vi "Cycle.vi"(8 "error in (no error)":errorcluster, 11 "WhiteNoiseOrientationDetection In":refnum<class "WhiteNoiseOrientationDetection.lvclass">) -> (0 "error out":errorcluster, 3 "WhiteNoiseOrientationDetection Out":refnum<class "WhiteNoiseOrientationDetection.lvclass">)   [LabVIEW 2014, in "WhiteNoiseOrientationDetection.lvclass"]
uses:
  WhiteNoiseOrientationDetection.lvclass
  WhiteNoiseOrientationDetection.lvclass/WhiteNoiseOrientationDetection.ctl
  Trial Based Experiment Statechart/MatlabExperiment/MatlabExperiment.lvclass
panel:
  in  "Override location":bool
  in  "location":dbl=1.0 max=10000.0
  in  "ExtraReward":dbl=0.8 min=0.0 step=0.1 format="%.1g"
  in  "Intertrial":dbl=1300.0
  in  "Override Coherence":bool
  in  "Override Signal":bool
  in  "Override Catch Trial":bool
  in  "coherence":dbl=35.0 max=10000.0
  in  "signal":dbl=135.0 max=10000.0
  in  "Override Timing":bool
  in  "PunishTime":dbl=2900.0
  out "InResponseWindow":bool
  in  "targetFixationRadius":dbl=75.0
  in  "nFramesCohTrain":dbl=50.0
  in  "nFramesPreMaxTrain":dbl=400.0
  in  "nFramesPreMeanTrain":dbl=150.0
  in  "nFramesPreMinTrain":dbl=100.0
  in  "responseIntervalTrain":dbl=50.0 max=10000.0
  in  "Eye Params":dbl[](array[numeric])
  out "XY Graph":cluster{dbl[], dbl[]}(graph)
  in  "MinReward":dbl=35.0
  in  "FixationRadius":dbl=50.0
  out "Timeouts":T1={"Intertrial"=1000.0, "AcquireFixation"=1000.0, "HoldFixation"=300.0, "DelayPeriod"=1000.0, "ResponsePeriod"=1000.0}
  out "ExperimentStats":T2
  out "Cycles":dbl
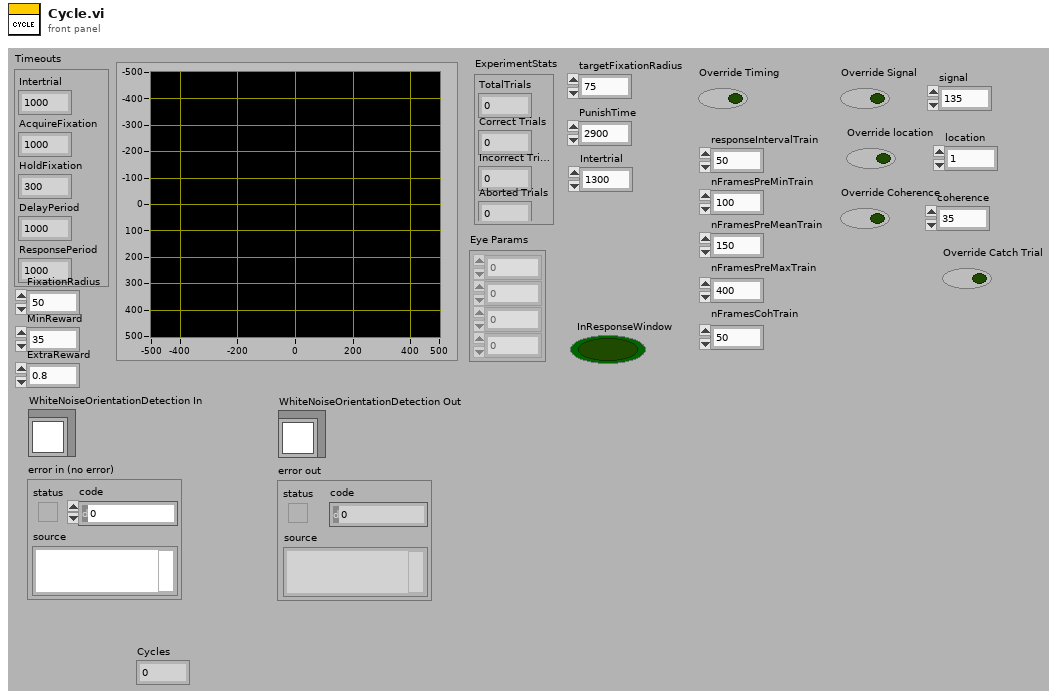
[diagram p1: front panel]
types:
  T1 = cluster{"Intertrial":dbl, "AcquireFixation":dbl, "HoldFixation":dbl, "DelayPeriod":dbl, "ResponsePeriod":dbl}
  T2 = cluster{"TotalTrials":dbl, "Correct Trials":dbl, "Incorrect Trials":dbl, "Aborted Trials":dbl}
  T3 = cluster{"TotalTrials":u32, "Correct Trials":u32, "Incorrect Trials":u32, "Aborted Trials":u32}
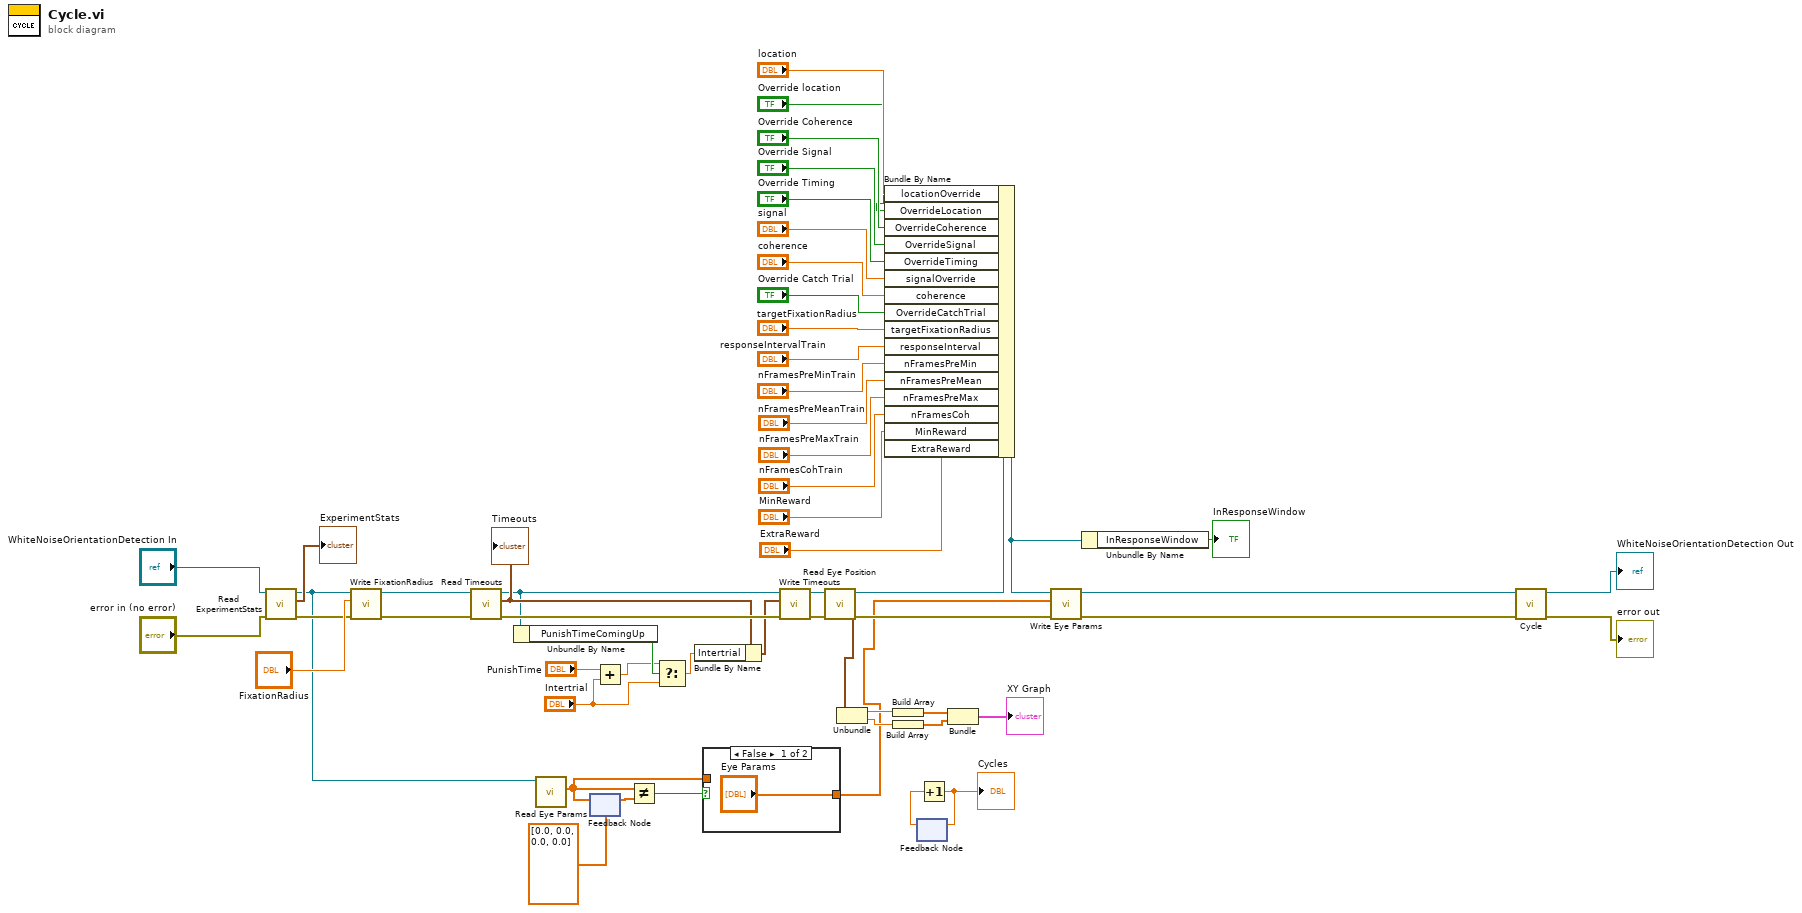
[diagram p0: block diagram]
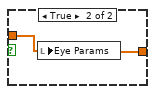
[diagram p2: hidden frame]
diagram:
  n1 = call-dynamic "Read ExperimentStats.vi"("error in (no error)"="error in (no error)", "TrialBasedExperiment in"="WhiteNoiseOrientationDetection In") -> ("error out"=w52:errorcluster, "ExperimentStats"=→"ExperimentStats":T3, "TrialBasedExperiment out"=w44:refnum<class "WhiteNoiseOrientationDetection.lvclass">)  [unwired: 7 in]
  n2 = call-dynamic "Write FixationRadius.vi"("error in (no error)"=w52, "FixationRadius"="FixationRadius", "MatlabExperiment in"=w44) -> ("error out"=w3:errorcluster, "MatlabExperiment out"=w4:refnum<class "WhiteNoiseOrientationDetection.lvclass">)  [unwired: 7 in]
  n3 = call-dynamic "Read Timeouts.vi"("error in (no error)"=w3, "TrialBasedExperiment in"=w4) -> ("error out"=w18:errorcluster, "Timeouts"=w15:T1, "TrialBasedExperiment out"=w12:refnum<class "WhiteNoiseOrientationDetection.lvclass">)  [unwired: 7 in]
  "Timeouts" <- w15
  n4 = Unbundle By Name(w12) -> ("PunishTimeComingUp"=w11:bool)
  n5 = call-dynamic "Read Eye Params.vi"("TrialBasedExperiment in"=w44) -> ("Eye Params"=w41:dbl[])  [unwired: 8 in, 2 out]
  n6 = feedback #1(dbl[] [0.0, 0.0, 0.0, 0.0] ("Eye Params")) -> (w43:dbl[])
  n7 = feedback-in #1(w41) -> ()
  n8 = Add(x="PunishTime", y="Intertrial") -> (x+y=w9:dbl)
  n9 = Not Equal?(x=w41, y=w43) -> (x != y?=w42:bool)
  n10 = Select(t=w9, s=w11, f="Intertrial") -> (s? t:f=w7:dbl)
  n11 = Bundle By Name(cluster=w15, "Intertrial"=w7) -> (w14:T1)
  n12 = case shown="False" w42 {
    tunnel: w41 -> [_ w58]
    tunnel: ["Eye Params" w58] -> w40
    frame False {
    }
    frame True {
      n13 = local write "Eye Params"(w58) -> ()
    }
  }
  n14 = call-dynamic "Write Timeouts.vi"("error in (no error)"=w18, "Timeouts"=w14, "TrialBasedExperiment in"=w12) -> ("error out"=w17:errorcluster, "TrialBasedExperiment out"=w16:refnum<class "WhiteNoiseOrientationDetection.lvclass">)  [unwired: 7 in]
  n15 = call-dynamic "Read Eye Position.vi"("error in (no error)"=w17, "TrialBasedExperiment in"=w16) -> ("error out"=w45:errorcluster, "Eye Position"=w51:cluster{"Horizontal":dbl, "Vertical":dbl}, "TrialBasedExperiment out"=w34:refnum<class "WhiteNoiseOrientationDetection.lvclass">)  [unwired: 7 in]
  n16 = Unbundle(w51) -> ("Horizontal"=w50:dbl, "Vertical"=w49:dbl)
  n17 = Bundle By Name(cluster=w34, "locationOverride"="location", "OverrideLocation"="Override location", "OverrideCoherence"="Override Coherence", "OverrideSignal"="Override Signal", "OverrideTiming"="Override Timing", "signalOverride"="signal", "coherence"="coherence", "OverrideCatchTrial"="Override Catch Trial", "targetFixationRadius"="targetFixationRadius", "responseInterval"="responseIntervalTrain", "nFramesPreMin"="nFramesPreMinTrain", "nFramesPreMean"="nFramesPreMeanTrain", "nFramesPreMax"="nFramesPreMaxTrain", "nFramesCoh"="nFramesCohTrain", "MinReward"="MinReward", "ExtraReward"="ExtraReward") -> (w27:refnum<class "WhiteNoiseOrientationDetection.lvclass">)
  n18 = Build Array(w50) -> (w48:dbl[])
  n19 = Build Array(w49) -> (w47:dbl[])
  n20 = feedback #2() -> (w55:dbl)  [unwired: 1 in]
  n21 = Increment(x=w55) -> (x+1=w56:dbl)
  "Cycles" <- w56
  n22 = feedback-in #2(w56) -> ()
  n23 = Bundle(w48, w47) -> (→"XY Graph":cluster{dbl[], dbl[]})  [unwired: 1 in]
  n24 = call-dynamic "Write Eye Params.vi"("error in (no error)"=w45, "Eye Params"=w40, "TrialBasedExperiment in"=w27) -> ("error out"=w25:errorcluster, "TrialBasedExperiment out"=w13:refnum<class "WhiteNoiseOrientationDetection.lvclass">)  [unwired: 7 in]
  n25 = Unbundle By Name(w27) -> ("InResponseWindow"=→"InResponseWindow":bool)
  n26 = call-parent "Cycle.vi"("error in (no error)"=w25, "MatlabExperiment In"=w13) -> ("error out"=→"error out":errorcluster, "MatlabExperiment Out"=→"WhiteNoiseOrientationDetection Out":refnum<class "WhiteNoiseOrientationDetection.lvclass">)  [unwired: 8 in]
